vi "Transceiver Thread.Transfer.Parse.vi"(8 "error in (no error)":errorcluster, 10 "Transfer":refnum<class "Transfer.lvclass">, 11 "Transceiver Thread in":refnum<class "Transceiver Thread.lvclass">) -> (0 "error out":errorcluster, 3 "Transceiver Thread out":refnum<class "Transceiver Thread.lvclass">)   [LabVIEW 2017, in "DSF Core.lvlib" / "Transceiver Thread.lvclass"]
uses:
  Transceiver Thread.lvclass
  Transfer/Transfer.lvclass
  Transceiver Thread.lvclass/Transceiver Thread.ctl
  Transfer/Transfer.lvclass/Transfer.ctl
  Buffer/Buffer.lvclass
  Pointer/DBL Pointer.lvclass
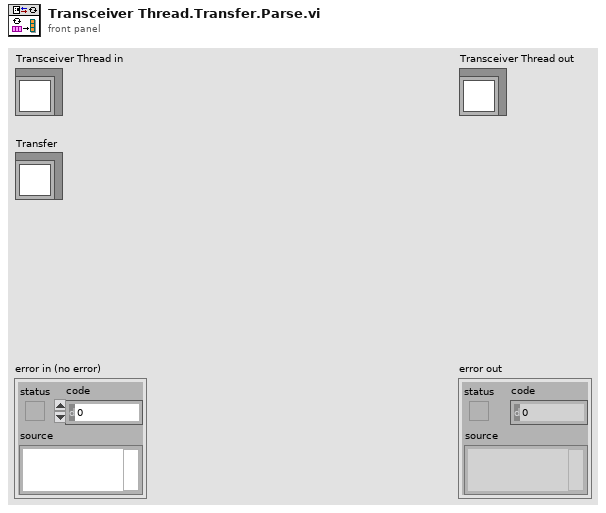
[diagram p1: front panel]
types:
  T1 = typedef "DSF Core.lvlib/DSF Runtime Type Buffers.ctl" = cluster{"Bool":bool[], "SGL":sgl[], "DBL":dbl[], "I8":i8[], "I16":i16[], "I32":i32[], "I64":i64[], "U8":u8[], "U16":u16[], "U32":u32[], "U64":u64[]}
  T2 = typedef "DSF Core.lvlib/DSF Runtime Channel Block.ctl" = cluster{"data type":T3, "count":u64, "buffer offset":u64}
  T3 = typedef "DSF Core.lvlib/Configuration.lvclass/DSF Data Type.ctl" = enum8{"Bool", "SGL", "DBL", "I8", "I16", "I32", "I64", "U8", "U16", "U32", "U64"}
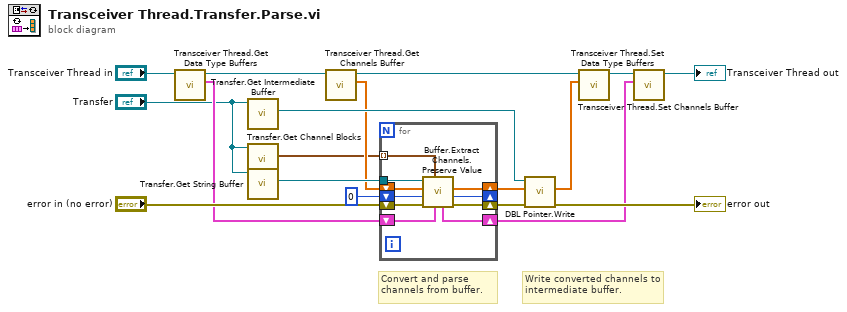
[diagram p0: block diagram]
diagram:
  # "Write converted channels to intermediate buffer."
  # "Convert and parse channels from buffer."
  n1 = call "Transceiver Thread.Get Data Type Buffers.vi"("Transceiver Thread in"="Transceiver Thread in") -> ("data type buffers"=w9:T1, "Transceiver Thread out"=w5:refnum<class "Transceiver Thread.lvclass">)  [unwired: 9 in]
  n2 = call "Transfer.Get Intermediate Buffer.vi"("Transfer in"="Transfer") -> ("DBL Buffer"=w14:refnum<class "DBL Pointer.lvclass">)  [unwired: 9 in, 1 out]
  n3 = call "Transfer.Get Channel Blocks.vi"("Transfer in"="Transfer") -> ("channel blocks"=w2:T2[])  [unwired: 9 in, 1 out]
  n4 = call "Transfer.Get String Buffer.vi"("Transfer in"="Transfer") -> ("Buffer"=w17:refnum<class "Buffer.lvclass">)  [unwired: 9 in, 1 out]
  n5 = call "Transceiver Thread.Get Channels Buffer.vi"("Transceiver Thread in"=w5) -> ("channels buffer"=w12:dbl[], "Transceiver Thread out"=w10:refnum<class "Transceiver Thread.lvclass">)  [unwired: 9 in]
  n6 = for {
    shift-right: [w27] -> w15
    shift-left: w12 -> [w25]
    shift-right: [w28] -> w16
    shift-left: "error in (no error)" -> [w26]
    tunnel: w17 -> [w24]
    tunnel: w2 -> [w21] mode=indexing
    shift-right: [w23] -> w8
    shift-left: w9 -> [w22]
    shift-right: [w20] -> _
    shift-left: u64 0 ("channels buffer index in") -> [w19]
    n7 = call "Buffer.Extract Channels.Preserve Value.vi"("data type buffers in"=w22, "channel block"=w21, "error in (no error)"=w26, "channels buffer index in"=w19, "channels buffer in"=w25, "Buffer in"=w24) -> ("error out"=w28:errorcluster, "channels buffer index out"=w20:u64, "channels buffer out"=w27:dbl[], "data type buffers out"=w23:T1)  [unwired: 1 in, 1 out]
  }
  n8 = call "DBL Pointer.Write.vi"("error in (no error)"=w16, "buffer in"=w15, "DBL Pointer in"=w14) -> ("error out"=→"error out":errorcluster, "buffer out"=w11:dbl[])  [unwired: 6 in, 1 out]
  n9 = call "Transceiver Thread.Set Channels Buffer.vi"("channels buffer"=w11, "Transceiver Thread in"=w10) -> ("Transceiver Thread out"=w4:refnum<class "Transceiver Thread.lvclass">)  [unwired: 9 in]
  n10 = call "Transceiver Thread.Set Data Type Buffers.vi"("data type buffers"=w8, "Transceiver Thread in"=w4) -> ("Transceiver Thread out"=→"Transceiver Thread out":refnum<class "Transceiver Thread.lvclass">)  [unwired: 9 in]
